vi "main_front_panel.vi"(0 "heat_board_control.lvclass":refnum<class "heat_board_control.lvclass">, 3 "manual setpoint voltage":dbl=0.825, 11 "PID":cluster{"P":dbl, "I":dbl, "D":dbl}={"P"=0.6, "I"=0.17, "D"=0.0}, 12 "LOCK":bool=TRUE, 14 "stop":bool) -> ()   [LabVIEW 2015]
uses:
  heat_board_control.lvclass
  Control 1.ctl
  magnetometer.lvclass
  <vilib>/DAQmx/read.llb/DAQmx Read (Analog Wfm 1Chan NSamp).vi
  global_stop_calibration.vi
  <vilib>/DAQmx/miscellaneous.llb/DAQmx Fill In Error Info.vi
  lock-in reference global.vi
panel:
  in  "Multicolumn Listbox":i32(listbox)=2
  in  "Tab Control":T1(tab)=enum."Stabilize Temperature"
  out "Sensor Status":string="\r\n"
  in  "COMM":refnum<visa-resource-name>="COM8"
  in  "Cluster":T3={"modulation_source"=enum."External", "Mode"=enum."Manual", "b2_field_offset"=0.0, "b1_field_offset"=0.0, "m2-field_offset"=0.0, "m1-field_offset"=0.0, "m2_mod_amp"=0.0, "m1-mod_amp"=0.0, "m2-analog_in"=FALSE, "m1-analog_in"=FALSE, "m2-filters"=FALSE, "m1-filters"=FALSE, "m2-lock"=FALSE, "m1-lock"=FALSE, "m2-modulation"=FALSE, "m1-modulation"=FALSE, "internal_mod_freq"=0.0, "external_mod_gain"=0.0, "m1-mod_phase"=1.0, "m2-mod_phase"=1.0, "m1-lock_output_gain"=0.0, "m2-lock_output_gain"=0.0, "m1-prop_gain"=0.0, "m2-prop_gain"=0.0, "m1-int_gain"=0.0, "m2-int_gain"=0.0, "m1-pid_gain"=0.0, "m2-pid_gain"=0.0, "m1-pid_output_gain"=0.0, "m2-pid_output_gain"=0.0, "m1-pid_inverse"=FALSE, "m2-pid_inverse"=FALSE} {"m2-mod_phase" min=1.0 max=30.0 step=1.0; "m1-mod_phase" min=1.0 max=30.0 step=1.0}
  out "Error Out":errorcluster={"status"=TRUE, "code"=-1073807339, "source"="VISA Read in serial_read_convert (SubVI).vi->NIST Labview UI R2.vi"}
  in  "restart averaging":bool
  in  "averaging parameters":T4={"averaging mode"=enum."No averaging", "weighting mode"=enum."Exponential", "number of averages"=10} {"number of averages" min=1}
  out "difference":cluster{"f0":dbl, "df":dbl, "magnitude":dbl[]}(graph)
  out "mag 2 data":cluster{"f0":dbl, "df":dbl, "magnitude":dbl[]}(graph)
  out "mag 1 data":cluster{"f0":dbl, "df":dbl, "magnitude":dbl[]}(graph)
  in  "magnetometer.lvclass":refnum<class "magnetometer.lvclass">
  in  "heat laser":u16(ring) items=["0", "1", "2", "3", "4", "5", "6", "7", "8", "9", "10", "11", "12", "13", "14", "15", "16", "17", "18", "19", "20", "21", "22", "23", "24", "25", "26", "27", "28", "29", "30", "31", "32", "33", "34", "35", "36", "37", "38", "39", "40", "41", "42", "43", "44", "45", "46", "47"]
  out "photodiode":dbl(graph)
  out "setpoint voltage (0V - 2V)":dbl(graph)
  in  "start1":bool
  in  "sampling info":cluster{"Fs":dbl, "#s":dbl}={"Fs"=5000.0, "#s"=500.0} {"Fs" format="%.2p"}
  out "locked":bool[](array[boolean])=[TRUE]
  out "XY Graph 2":cluster{"X":dbl, "Y":dbl}[](graph)
  in  "heat laser select":u16(ring) items=["0", "1", "2", "3", "4", "5", "6", "7", "8", "9", "10", "11", "12", "13", "14", "15", "16", "17", "18", "19", "20", "21", "22", "23", "24", "25", "26", "27", "28", "29", "30", "31", "32", "33", "34", "35", "36", "37", "38", "39", "40", "41", "42", "43", "44", "45", "46", "47"]
  in  "OK Button":bool
  in  "end":bool
  in  "lock-in reference channel":tag="PXI1Slot4/ai2"
  in  "start2":bool
  out "Percent Done":dbl(knob) scale=0.0..100.0
  in  "database connection":path=path "O:/ADI/nardelli/TMS_nn/sensor_defaults.udl"
  in  "stop 2":bool caption="stop"
  out "Running":bool=TRUE
  # "select magnetometers and cells to run"
  # "Communicate with the QuSpin box.  Change the numeric controls and click the buttons to change the state of the QuSpin box."
  # "Modulation Source"
  # "Internal Modulation Frequency (0.01Hz - 24kHz)"
  # "External Modulation Gain (0 - 15.9999)"
  # "B 1"
  # "B 2"
  # "Field Offset"
  # "Mag 1"
  # "Mag 2"
  # "Modulation"
  # "Lock"
  # "Filters"
  # "Analog Output\n(PID / Lock-in)"
  # "Modulation\nGain"
  # "DC Field Offset"
  # "Modulation Phase (1-30)"
  # "Lock-in Output Gain (0 - 15.9999)"
  # "Proportional Gain (0 - 15.9999)"
  # "Integral Gain (0 - 15.9999)"
  # "PID Gain (0 - 15.9999)"
  # "PID Output Gain (0 - 15.9999)"
  # "PID Inverse"
  # "Stabilize each rubidium cell to its most sensitive temperature.  Set the proper PID parameters as well as the ADC sampling parameters.  Click \"START\" and then \"LOCK\" to start the feedback loop for all connected cells.  The photodiode will reach its setpoint (most sensitive cell temperature) and then the system will be ready to take magnetic data."
  # "Start/Stop and lock all lasers"
  # "monitor the photodiode and setpoint of a specific laser"
  # "Set up the heat lasers.  Select the input/output related to each heat laser and make sure the database connection is pointed to the correct database.  Clicking \"START\" will start the calibration of each of the selected heat lasers.  You will see the progress as each heat laser finds its most sensitive temperature and once this process is complete, each temperature is saved in the database for easy retreival by the temperature stabilization loop."
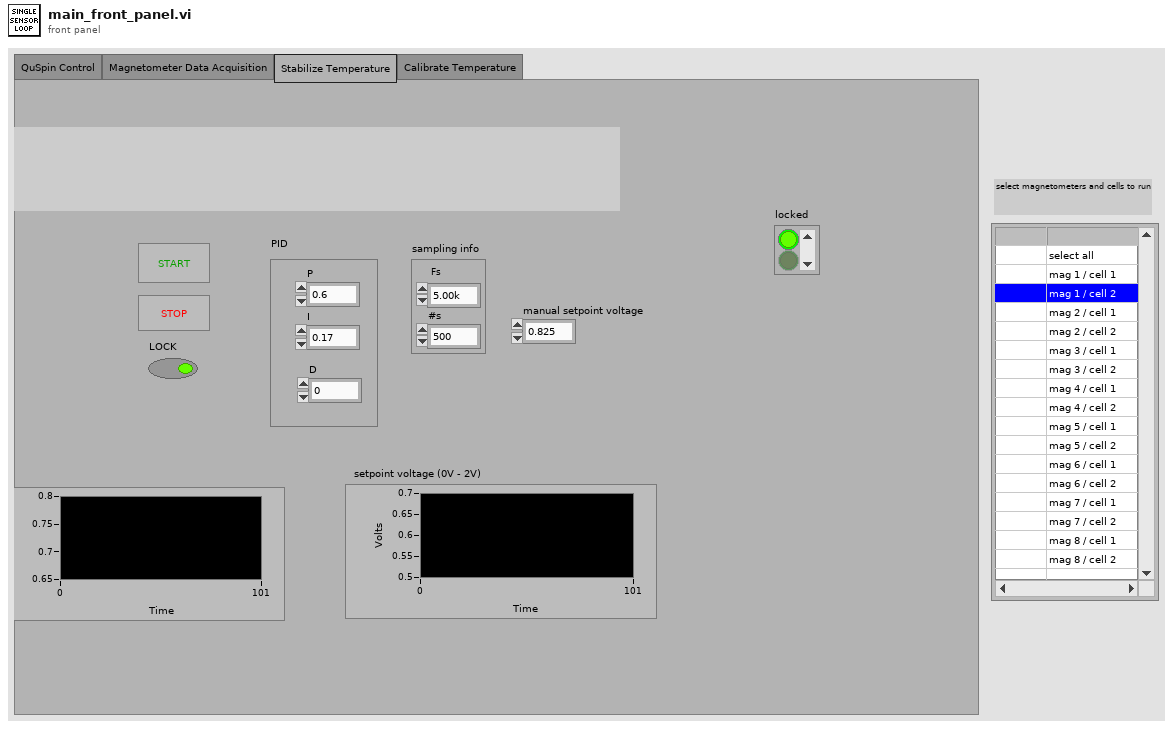
[diagram p1: front panel]
types:
  T1 = enum32{"QuSpin Control", "Magnetometer Data Acquisition", "Stabilize Temperature", "Calibrate Temperature"}
  T2 = typedef "Control 1.ctl" = dbl
  T3 = cluster{"modulation_source":enum32{"External", "Internal"}, "Mode":enum32{"Manual", "TTL"}, "b2_field_offset":dbl, "b1_field_offset":dbl, "m2-field_offset":dbl, "m1-field_offset":dbl, "m2_mod_amp":dbl, "m1-mod_amp":dbl, "m2-analog_in":bool, "m1-analog_in":bool, "m2-filters":bool, "m1-filters":bool, "m2-lock":bool, "m1-lock":bool, "m2-modulation":bool, "m1-modulation":bool, "internal_mod_freq":dbl, "external_mod_gain":dbl, "m1-mod_phase":T2, "m2-mod_phase":dbl, "m1-lock_output_gain":dbl, "m2-lock_output_gain":dbl, "m1-prop_gain":dbl, "m2-prop_gain":dbl, "m1-int_gain":dbl, "m2-int_gain":dbl, "m1-pid_gain":dbl, "m2-pid_gain":dbl, "m1-pid_output_gain":dbl, "m2-pid_output_gain":dbl, "m1-pid_inverse":bool, "m2-pid_inverse":bool}
  T4 = cluster{"averaging mode":enum16{"No averaging", "Vector averaging", "RMS averaging", "Peak hold"}, "weighting mode":enum16{"Linear", "Exponential"}, "number of averages":u32}
  T5 = cluster{string, "DAQmx Physical Channel":tag, "physical channel":refnum<k21>, "DAQmx Physical Channel":tag}[]
  T6 = cluster{"DAQmx Physical Channel":tag, "DAQmx Physical Channel":tag}[]
  T7 = cluster{"modulation_source":bool, "Mode":bool, "b2_field_offset":bool, "b1_field_offset":bool, "m2-field_offset":bool, "m1-field_offset":bool, "m2_mod_amp":bool, "m1-mod_amp":bool, "m2-analog_in":bool, "m1-analog_in":bool, "m2-filters":bool, "m1-filters":bool, "m2-lock":bool, "m1-lock":bool, "m2-modulation":bool, "m1-modulation":bool, "internal_mod_freq":bool, "external_mod_gain":bool, "m1-mod_phase":bool, "m2-mod_phase":bool, "m1-lock_output_gain":bool, "m2-lock_output_gain":bool, "m1-prop_gain":bool, "m2-prop_gain":bool, "m1-int_gain":bool, "m2-int_gain":bool, "m1-pid_gain":bool, "m2-pid_gain":bool, "m1-pid_output_gain":bool, "m2-pid_output_gain":bool, "m1-pid_inverse":bool, "m2-pid_inverse":bool}
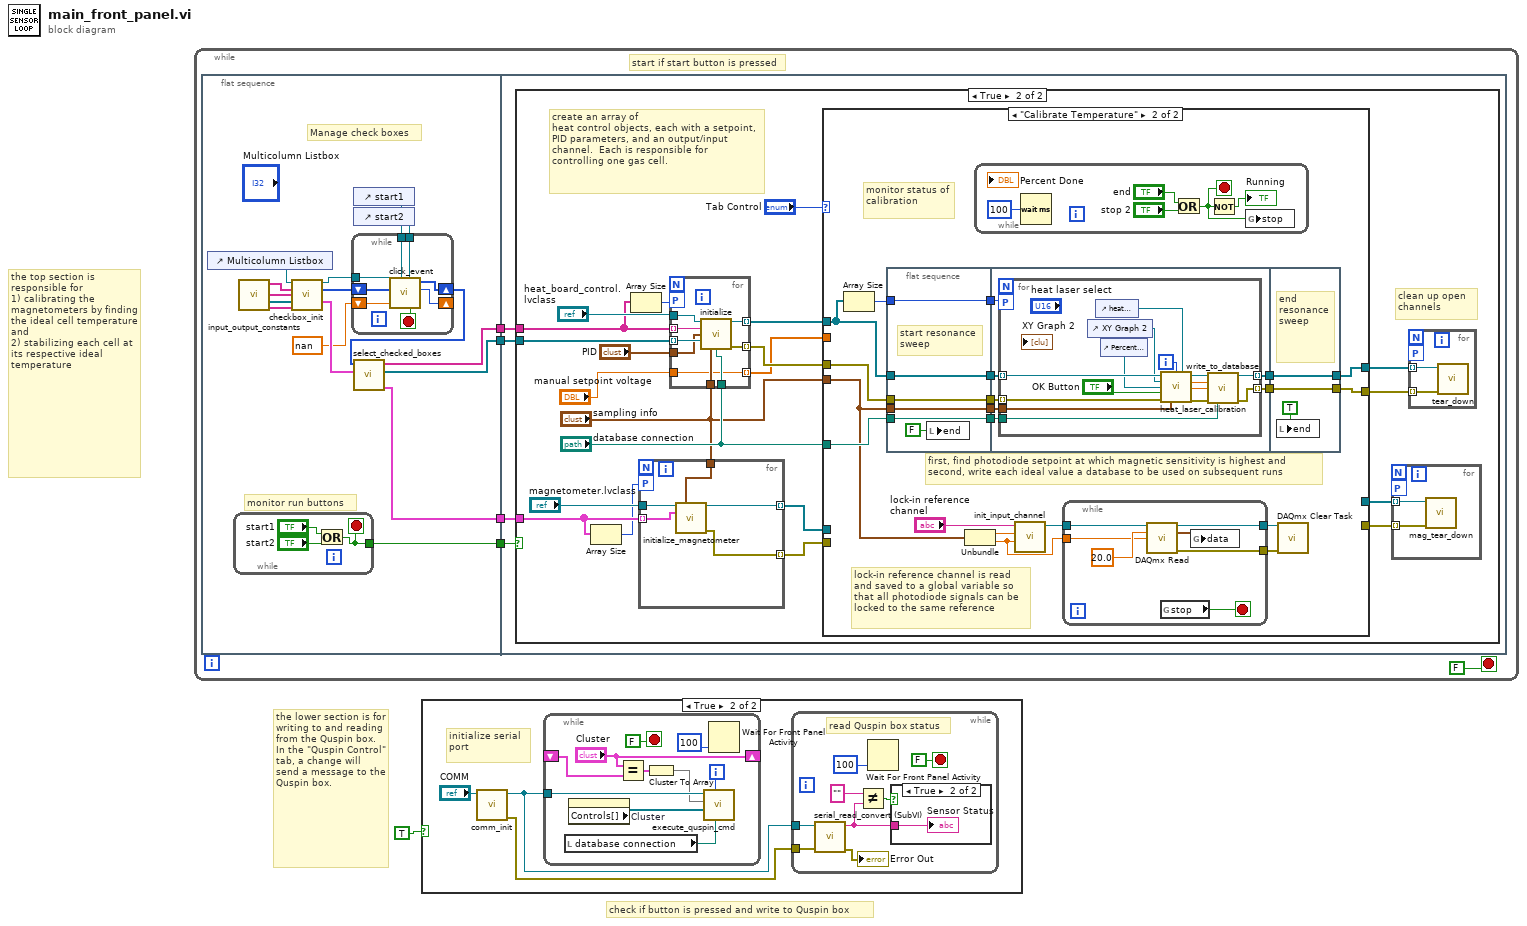
[diagram p0: block diagram]
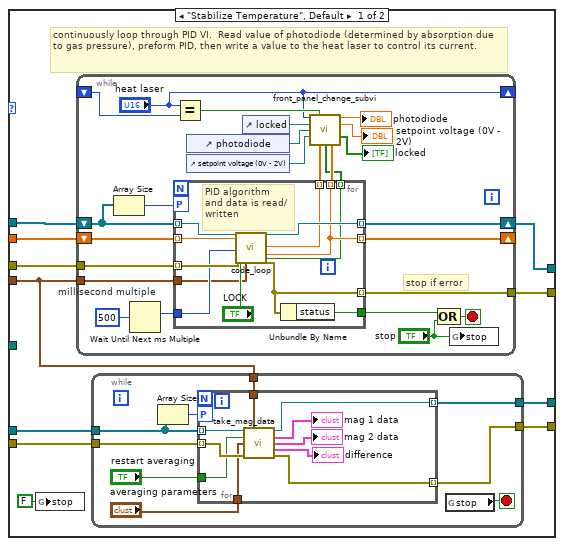
[diagram p5: hidden frame]
diagram:
  # "check if button is pressed and write to Quspin box"
  # "the top section is responsible for  \n1) calibrating the magnetometers by finding the ideal cell temperature and \n2) stabilizing each cell at its respective ideal temperature"
  # "the lower section is for writing to and reading from the Quspin box.  In the \"Quspin Control\" tab, a change will send a message to the Quspin box."
  n1 = while {
    stop <- FALSE stop-if-true
    # "start if start button is pressed"
    n2 = flat-sequence {
      tunnel: [w22] -> w5
      tunnel: [w9] -> w4
      tunnel: [w8] -> w3
      tunnel: [w7] -> w2
      tunnel: w5 -> [w37]
      tunnel: w4 -> [w36]
      tunnel: w3 -> [w35]
      tunnel: w2 -> [w34]
      frame #0 {
        # "monitor run buttons"
        # "Manage check boxes"
        n3 = control-ref of="Multicolumn Listbox"() -> (w15:refnum<vi>)
        n4 = while {
          tunnel: [w23] -> w22
          stop <- w23 stop-if-true
          n5 = Or(x="start1", y="start2") -> (x .or. y?=w23:bool)
        }
        n6 = call "input_output_constants.vi"() -> ("mag inputs"=w19:tag[], "heat outputs"=w20:refnum<k21>[], "heat inputs"=w21:tag[], "labels"=w13:string[])  [unwired: 8 in]
        n7 = call "checkbox_init.vi"("MulticolumnListbox in"=w15, "labels"=w13, "heat inputs"=w21, "heat outputs"=w20, "mag inputs"=w19) -> ("MulticolumnListbox out"=w16:refnum<vi>, "checkbox array"=w14:i32[], "i/o array"=w17:T5)  [unwired: 8 in]
        n8 = control-ref of="start1"() -> (w11:refnum<vi>)
        n9 = control-ref of="start2"() -> (w10:refnum<vi>)
        n10 = while {
          shift-right: [w29] -> _
          shift-left: nan -> [w31]
          shift-right: [w30] -> w18
          shift-left: w14 -> [w32]
          tunnel: w16 -> [w33]
          tunnel: w10 -> [w28]
          tunnel: w11 -> [w27]
          stop <- w26 stop-if-true
          n11 = call "click_event.vi"("start2 2"=w28, "start1 2"=w27, "focus row"=w31, "checkbox array in"=w32, "MulticolumnListbox in"=w33) -> ("Boolean"=w26:bool, "FocusRow"=w29:i32, "checkbox array out"=w30:i32[])  [unwired: 4 in]
        }
        n12 = call "select_checked_boxes.vi"("i/o array"=w17, "checkbox array"=w18) -> ("array of mag inputs"=w7:T6, "heat outputs"=w8:refnum<k21>[], "heat inputs"=w9:tag[])  [unwired: 6 in, 1 out]
      }
      frame #1 {
        n13 = case shown="True" w37 {
          tunnel: w36 -> [_ w41]
          tunnel: w35 -> [_ w51]
          tunnel: w34 -> [_ w39]
          frame False {
          }
          frame True {
            # "create an array of \nheat control objects, each with a setpoint, PID parameters, and an output/input channel.  Each is responsible for controlling one gas cell."
            # "clean up open \nchannels"
            n14 = Array Size(array=w39) -> (size(s)=w38:i32)
            n15 = Array Size(array=w41) -> (size(s)=w40:i32)
            n16 = for {
              tunnel: "magnetometer.lvclass" -> [w64]
              tunnel: "sampling info" -> [w65]
              tunnel: w39 -> [w63] mode=indexing
              tunnel: [w62] -> w46 mode=indexing
              tunnel: [w61] -> w45 mode=indexing
              workers-P: w38 -> [_]
              n17 = call-dynamic "initialize_magnetometer.vi"("magnetometer in"=w64, "sampling info"=w65, "mag inputs"=w63) -> ("magnetometer out"=w62:refnum<class "magnetometer.lvclass">, "error out"=w61:errorcluster)  [unwired: 11 in]
            }
            n18 = for {
              tunnel: w41 -> [w74] mode=indexing
              tunnel: w51 -> [w73] mode=indexing
              tunnel: "PID" -> [w72]
              tunnel: [w71] -> w58 mode=indexing
              tunnel: "heat_board_control.lvclass" -> [w70]
              tunnel: [w69] -> w57 mode=indexing
              workers-P: w40 -> [_]
              tunnel: "sampling info" -> [w68]
              tunnel: "database connection" -> [w67]
              tunnel: "manual setpoint voltage" -> [w66]
              tunnel: [w66] -> w49 mode=indexing
              n19 = call "initialize.vi"("heat_board_control in 2"=w70, "input channel"=w74, "PID"=w72, "output channel"=w73, "sampling info"=w68, "setpoint"=w67) -> ("heat_board_control out 2"=w69:refnum<class "heat_board_control.lvclass">, "error out"=w71:errorcluster)  [unwired: 8 in]
            }
            n20 = case shown="\"Calibrate Temperature\"" "Tab Control" {
              tunnel: [w85 w158] -> w54
              tunnel: [w84 w157] -> w53
              tunnel: w49 -> [w83 _]
              tunnel: "sampling info" -> [w80 w154]
              tunnel: w58 -> [w82 w160]
              tunnel: w57 -> [w81 w143]
              tunnel: "database connection" -> [_ w159]
              tunnel: w46 -> [w79 _]
              tunnel: w45 -> [w78 _]
              tunnel: [w77 _] -> w44
              tunnel: [w76 _] -> w43
              frame "Stabilize Temperature", Default {
                # "continuously loop through PID VI.  Read value of photodiode (determined by absorption due to gas pressure), preform PID, then write a value to the heat laser to control its current."
                n21 = global write "global_stop_calibration.vi" "stop"(FALSE ("stop")) -> ()
                n22 = while {
                  shift-right: [w121] -> w85
                  shift-left: w81 -> [w106]
                  tunnel: w82 -> [w127]
                  shift-right: [w126] -> _
                  shift-left: w83 -> [w128]
                  tunnel: [w125] -> w84
                  tunnel: w80 -> [w120]
                  shift-right: ["heat laser"] -> _
                  shift-left: _ -> [w109]
                  stop <- w123 stop-if-true
                  w122 = u32 500  # millisecond multiple
                  # "stop if error"
                  n23 = Array Size(array=w106) -> (size(s)=w105:i32)
                  n24 = Wait Until Next ms Multiple(millisecond multiple=w122) -> ()  [unwired: 1 out]
                  n25 = for {
                    tunnel: w106 -> [w140] mode=indexing
                    tunnel: w128 -> [w139] mode=indexing
                    tunnel: [w134] -> w126 mode=indexing
                    tunnel: [w136] -> w121 mode=indexing
                    tunnel: [w135] -> w116 mode=indexing
                    tunnel: [w134] -> w115 mode=indexing
                    tunnel: [w133] -> w114 mode=indexing
                    tunnel: w127 -> [w137] mode=indexing
                    tunnel: [w132] -> w125 mode=indexing
                    tunnel: [w131] -> w124
                    tunnel: w122 -> [w130]
                    workers-P: w105 -> [_]
                    tunnel: w120 -> [w129]
                    # "PID algorithm\nand data is read/\nwritten"
                    n26 = call-dynamic "code_loop.vi"("heat_board_control in"=w140, "laser setpoint in"=w139, "millisecond\n multiple"=w130, "lock all"="LOCK", "error in (no error)"=w137, "sampling info"=w129) -> ("heat_board_control out"=w136:refnum<class "heat_board_control.lvclass">, "data average"=w135:dbl, "laser setpoint out"=w134:dbl, "Boolean"=w133:bool, "error out"=w132:errorcluster)  [unwired: 16 in, 1 out]
                    n27 = Unbundle By Name(w132) -> ("status"=w131:bool)
                  }
                  n28 = Equal?(x="heat laser", y=w109) -> (x = y?=w111:bool)
                  n29 = control-ref of="photodiode"() -> (w113:refnum<vi>)
                  n30 = control-ref of="setpoint voltage (0V - 2V)"() -> (w112:refnum<vi>)
                  n31 = control-ref of="locked"() -> (w110:refnum<vi>)
                  n32 = call "front_panel_change_subvi.vi"("index"="heat laser", "Boolean"=w111, "locked reference"=w110, "PD reference"=w113, "setpoint voltage reference"=w112, "PD"=w116, "locked"=w114, "setpoint voltage"=w115) -> ("photodiode"=→"photodiode":dbl, "setpoint voltage (0V - 2V)"=→"setpoint voltage (0V - 2V)":dbl, "locked"=→"locked":bool[])  [unwired: 5 in]
                  n33 = Compound Arithmetic op=OR(w124, "stop") -> (w123:bool)
                  n34 = global write "global_stop_calibration.vi" "stop"("stop") -> ()
                }
                n35 = while {
                  tunnel: w80 -> [w93]
                  tunnel: w79 -> [w89]
                  tunnel: w78 -> [w94]
                  tunnel: [w92] -> w77
                  tunnel: [w91] -> w76
                  stop <- w90 stop-if-true
                  n36 = Array Size(array=w89) -> (size(s)=w88:i32)
                  n37 = for {
                    tunnel: w89 -> [w104] mode=indexing
                    tunnel: w94 -> [w103] mode=indexing
                    tunnel: w93 -> [w102]
                    tunnel: [w101] -> w92 mode=indexing
                    tunnel: [w100] -> w91 mode=indexing
                    workers-P: w88 -> [_]
                    tunnel: "restart averaging" -> [w96]
                    tunnel: "averaging parameters" -> [w95]
                    n38 = call-dynamic "take_mag_data.vi"("magnetometer in"=w104, "sampling info"=w102, "restart averaging"=w96, "averaging parameters"=w95, "error in (no error)"=w103) -> ("magnetometer out"=w101:refnum<class "magnetometer.lvclass">, "mag 1 data"=→"mag 1 data":cluster{"f0":dbl, "df":dbl, "magnitude":dbl[]}, "mag 2 data"=→"mag 2 data":cluster{"f0":dbl, "df":dbl, "magnitude":dbl[]}, "difference"=→"difference":cluster{"f0":dbl, "df":dbl, "magnitude":dbl[]}, "error out"=w100:errorcluster)  [unwired: 6 in]
                  }
                  n39 = global read "global_stop_calibration.vi" "stop"() -> (w90:bool)
                }
              }
              frame "Calibrate Temperature" {
                # "lock-in reference channel is read and saved to a global variable so that all photodiode signals can be locked to the same reference"
                # "first, find photodiode setpoint at which magnetic sensitivity is highest and \nsecond, write each ideal value a database to be used on subsequent runs"
                # "monitor status of calibration"
                n40 = Array Size(array=w143) -> (size(s)=w141:i32)
                n41 = flat-sequence {
                  tunnel: w154 -> [w163]
                  tunnel: w159 -> [w164]
                  tunnel: w160 -> [w165]
                  tunnel: w143 -> [w166]
                  tunnel: [w166] -> w147
                  tunnel: [w165] -> w146
                  tunnel: [w164] -> w145
                  tunnel: [w163] -> w144
                  tunnel: [w161] -> w142
                  tunnel: w141 -> [w161]
                  tunnel: [w170] -> w151
                  tunnel: [w169] -> w150
                  tunnel: w147 -> [w173]
                  tunnel: w146 -> [w172]
                  tunnel: w145 -> [w171]
                  tunnel: w144 -> [w168]
                  tunnel: w142 -> [w167]
                  tunnel: [w190] -> w157
                  tunnel: [w191] -> w158
                  tunnel: w151 -> [w191]
                  tunnel: w150 -> [w190]
                  frame #0 {
                    # "start resonance sweep"
                    n42 = local write "end"(FALSE) -> ()
                  }
                  frame #1 {
                    n43 = for {
                      tunnel: w168 -> [w184]
                      tunnel: w172 -> [w185] mode=indexing
                      tunnel: w171 -> [w176]
                      tunnel: w173 -> [w186] mode=indexing
                      tunnel: [w188] -> w170 mode=indexing
                      tunnel: [w187] -> w169 mode=indexing
                      workers-P: w167 -> [_]
                      i -> [w179]
                      n44 = control-ref of="XY Graph 2"() -> (w177:refnum<vi>)
                      n45 = control-ref of="heat laser select"() -> (w178:refnum<vi>)
                      n46 = control-ref of="Percent Done"() -> (w181:refnum<vi>)
                      n47 = call "heat_laser_calibration.vi"("heat_board_control.lvclass"=w186, "sampling info"=w184, "ID"=w179, "heat laser select"=w178, "XY Graph"=w177, "Percent Done"=w181, "error in (no error)"=w185, "first calibration"="OK Button") -> ("heat_board_control out"=w183:refnum<class "heat_board_control.lvclass">, "best setpoint"=w175:dbl, "best manual laser"=w174:dbl, "error out"=w182:errorcluster)  [unwired: 2 in, 2 out]
                      n48 = call "write_to_database.vi"("heat_board_control in"=w183, "best setpoint"=w175, "best manual laser"=w174, "error in (no error)"=w182, "database connection"=w176) -> ("heat_board_control out"=w188:refnum<class "heat_board_control.lvclass">, "error out"=w187:errorcluster)  [unwired: 9 in]
                    }
                  }
                  frame #2 {
                    # "end resonance sweep"
                    n49 = local write "end"(TRUE ("stop")) -> ()
                  }
                }
                n50 = Unbundle(w154) -> ("Fs"=w153:dbl, "#s"=w152:dbl)
                n51 = while {
                  stop <- w200 stop-if-true
                  n52 = Wait (ms)(milliseconds to wait=u32 100) -> ()  [unwired: 1 out]
                  n53 = Or(x="end", y="stop 2") -> (x .or. y?=w200:bool)
                  n54 = Not(x=w200) -> (.not. x?=→"Running":bool)
                  n55 = global write "global_stop_calibration.vi" "stop"(w200) -> ()
                }
                n56 = call "init_input_channel.vi"("samples per channel"=w152, "rate"=w153, "input channel"="lock-in reference channel") -> ("task out"=w156:refnum<k21>)  [unwired: 7 in, 1 out]
                n57 = while {
                  tunnel: w156 -> [w196]
                  tunnel: w152 -> [w195]
                  tunnel: [w194] -> w149
                  tunnel: [w193] -> w148
                  stop <- w192 stop-if-true
                  n58 = call-poly <vilib>:"DAQmx Read.vi"("task/channels in"=w196, "number of samples per channel"=w195, "timeout"=20.0) -> ("task out"=w194:refnum<k21>, "data"=w197:waveform(dbl), "error out"=w193:errorcluster)  [unwired: 10 in]
                  n59 = global read "global_stop_calibration.vi" "stop"() -> (w192:bool)
                  n60 = global write "lock-in reference global.vi" "data"(w197) -> ()
                }
                n61 = call <vilib>:"DAQmx Clear Task.vi"("task in"=w149, "error in"=w148) -> ()  [unwired: 13 in, 1 out]
              }
            }
            n62 = for {
              workers-P: _ -> [_]
              tunnel: w44 -> [w60] mode=indexing
              tunnel: w43 -> [w59] mode=indexing
              n63 = call-dynamic "mag_tear_down.vi"("error in (no error)"=w59, "magnetometer in"=w60) -> ()  [unwired: 8 in, 2 out]
            }
            n64 = for {
              tunnel: w54 -> [w205] mode=indexing
              tunnel: w53 -> [w204] mode=indexing
              workers-P: _ -> [_]
              n65 = call-dynamic "tear_down.vi"("error in (no error)"=w204, "heat_board_control in"=w205) -> ()  [unwired: 8 in, 2 out]
            }
          }
        }
      }
    }
  }
  n66 = case shown="True" TRUE {
    frame False {
    }
    frame True {
      # "initialize serial port"
      n67 = call "comm_init.vi"("VISA Refnum in"="COMM") -> ("error out"=w206:errorcluster, "VISA Refnum out"=w208:refnum<visa-resource-name>)  [unwired: 9 in]
      n68 = while {
        shift-right: ["Cluster"] -> _
        shift-left: _ -> [w227]
        tunnel: w208 -> [w223]
        i -> [w218]
        stop <- FALSE stop-if-true
        n69 = local read "database connection"() -> (w220:path)
        n70 = property on="Cluster" class="Clust (strict)"() -> ("Controls[]"=w219:refnum<vi>[])  [unwired: 2 in, 2 out]
        n71 = Equal?(x="Cluster", y=w227) -> (x = y?=w224:T7)
        n72 = Cluster To Array(cluster=w224) -> (array=w221:bool[])
        n73 = call "execute_quspin_cmd.vi"("database connection"=w220, "while loop index"=w218, "Controls[]"=w219, "Array"=w221, "VISA Refnum in"=w223) -> ()  [unwired: 7 in]
        n74 = Wait For Front Panel Activity(1:100 ("timeout ms (-1 never timeout)")) -> ()  [unwired: 2 in, 1 out]
      }
      n75 = while {
        tunnel: w208 -> [w213]
        tunnel: w206 -> [w210]
        stop <- FALSE stop-if-true
        # "read Quspin box status"
        n76 = call "serial_read_convert (SubVI).vi"("error in (no error)"=w210, "VISA Refnum in"=w213) -> ("error out"=→"Error Out":errorcluster, "read buffer All"=w212:string)  [unwired: 6 in, 2 out]
        n77 = Not Equal?(x="", y=w212) -> (x != y?=w216:bool)
        n78 = Wait For Front Panel Activity(1:100 ("timeout ms (-1 never timeout)")) -> ()  [unwired: 2 in, 1 out]
        n79 = case shown="True" w216 {
          tunnel: w212 -> [_ w217]
          frame False {
          }
          frame True {
            "Sensor Status" <- w217
          }
        }
      }
    }
  }
